vi "Elapsed_s.vi"(11 "Error in":errorcluster caption="Error in (no error)", 12 "Start time in":i64=-1 caption="Start time in (-1: init) [ms]" min=-1 max=4294967295) -> (8 "Elapsed time":dbl caption="Elapsed time [s]", 13 "Now":i64 caption="Now [ms]", 14 "Start time out":i64 caption="Start time out [ms]", 15 "Error out":errorcluster)   [LabVIEW 2017, in "GPTiming.lvlib"]
doc: "Calculates <B>Elapsed time</B> since <B>Start time in</B>.\n\n<B>Start time in</B> will be returned in <B>Start time out</B>. Set <B>Start time in</B> to -1 (or leave it unwired) to get the current time returned in <B>Start time out</B> instead. <B>Now</B> will always be the current time.\n\nThis VI uses the ms tick counter and will be able to count for 2^32-1 ms (almost 50 days) before <B>Elapsed time</B> wraps around and starts from zero again.\n\nThis VI is inlined. <B>Error in</B> is wired straight through to <B>Error out</B> to enable optional dataflow dependency (offering control of when <B>Now</B> is).\n\nSteen Schmidt\nGPower\n8/12 2013"
uses:
  GPTiming.lvlib
panel:
  # "Copyright © 2013\nGPower\nSee enclosed license file for terms and conditions"
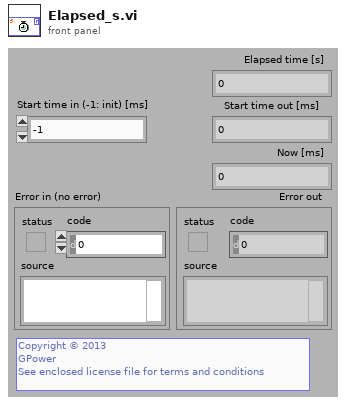
[diagram p1: front panel]
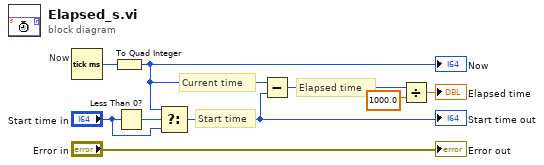
[diagram p0: block diagram]
diagram:
  # "Elapsed time"
  # "Current time"
  # "Start time"
  n1 = Tick Count (ms) "Now"() -> (millisecond timer value=w4:u32)
  n2 = To Quad Integer(1:w4) -> (0:w5:i64)
  "Now" <- w5
  n3 = Less Than 0?(x="Start time in") -> (x < 0?=w9:bool)
  n4 = Select(t=w5, s=w9, f="Start time in") -> (s? t:f=w6:i64)
  "Start time out" <- w6
  n5 = Subtract(x=w5, y=w6) -> (x-y=w3:i64)
  n6 = Divide(x=w3, y=1000.0) -> (x/y=→"Elapsed time":dbl)
  "Error out" <- "Error in"
